vi "class_data.vi"() -> ()   [LabVIEW 2010, in "TrajectoryMH100122AODRAPS.lvclass"]
uses:
  TrajectoryMH100122AODRAPS.lvclass
  common/xcontrols/XImage/XImage/XImage.xctl
panel:
  in  "XImage reference":refnum<vi>
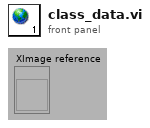
[diagram p1: front panel]
diagram:
